vi "Gen - Get Font List.vi"(8 "Error In":errorcluster) -> (0 "Error Out":errorcluster, 3 "Font List":string[](array[string]))   [LabVIEW 2020]
uses:
  <vilib>/registry/registry.llb/Registry RtKey.ctl
  <vilib>/registry/registry.llb/Registry SAM.ctl
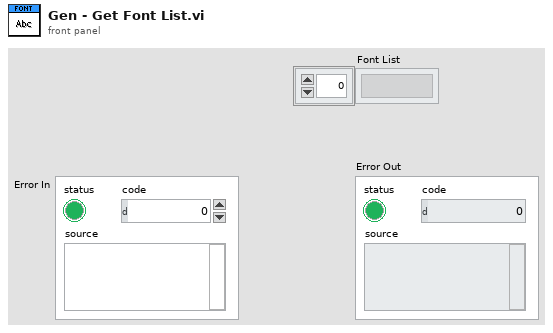
[diagram p1: front panel]
types:
  T1 = typedef "Registry SAM.ctl" = enum32{"KEY_QUERY_VALUE", "KEY_SET_VALUE", "KEY_CREATE_SUB_KEY", "KEY_ENUMERATE_SUB_KEYS", "KEY_NOTIFY", "KEY_CREATE_LINK", "KEY_READ", "KEY_WRITE", "KEY_ALL_ACCESS", "KEY_READ | KEY_WRITE"}
  T2 = typedef "Registry RtKey.ctl" = enum32{"HKEY_CLASSES_ROOT", "HKEY_CURRENT_USER", "HKEY_LOCAL_MACHINE", "HKEY_USERS", "HKEY_PERFORMANCE_DATA", "HKEY_CURRENT_CONFIG", "HKEY_DYN_DATA"}
  T3 = typedef "Registry refnum.ctl" = refnum<k1>
  T4 = cluster{"numValues":i32, "maxValueNameLen":i32, "maxValueDataLen":i32}
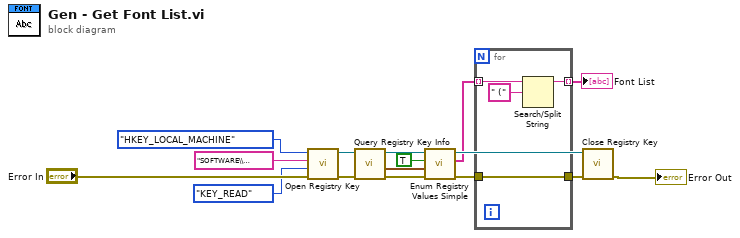
[diagram p0: block diagram]
diagram:
  n1 = call <vilib>:"Open Registry Key.vi"("error in (no error)"="Error In", "security access mask (KEY_READ | KEY_WRITE)"=Registry_SAM."KEY_READ", "subkey"="SOFTWARE\\Microsoft\\Windows NT\\CurrentVersion\\Fonts\\", "root key (HKEY_LOCAL_MACHINE)"=Registry_RtKey."HKEY_LOCAL_MACHINE") -> ("error out"=w16:errorcluster, "refnum out"=w8:T3)  [unwired: 6 in]
  n2 = call <vilib>:"Query Registry Key Info.vi"("error in (no error)"=w16, "refnum"=w8) -> ("error out"=w15:errorcluster, "value info"=w4:T4, "refnum out"=w6:T3)  [unwired: 5 in, 2 out]
  n3 = call <vilib>:"Enum Registry Values Simple.vi"("error in (no error)"=w15, "value info"=w4, "retrieve data? (F)"=TRUE, "refnum"=w6) -> ("error out"=w13:errorcluster, "values"=w2:string[], "refnum out"=w5:T3)  [unwired: 2 in, 3 out]
  n4 = for {
    tunnel: w2 -> [w19] mode=indexing
    tunnel: [w17] -> w1 mode=indexing
    tunnel: [w20] -> w14
    tunnel: w13 -> [w20]
    n5 = Search/Split String(string=w19, search string/char (-)=" (") -> (substring before match=w17:string)  [unwired: 1 in, 2 out]
  }
  "Font List" <- w1
  n6 = call <vilib>:"Close Registry Key.vi"("error in (no error)"=w14, "refnum"=w5) -> ("error out"=→"Error Out":errorcluster)  [unwired: 5 in]
